vi "Menu.Sequeunce.Execute.vi"(8 "error in (no error)":errorcluster, 9 "Coords":T1, 10 "ItemPath":string, 11 "State Variables":T2={"Aliases.All"=[], "Aliases.Outputs"=[], "UI.Sequence#ofColumns"=0, "SysDef.Path"=path "", "UI.SequenceRef"=refnum, "UI.StepInformationRef"=refnum, "UI.AbortRef"=refnum, "UI.GraphRef"=refnum, "UI.ViewRef"=refnum, "UI.IterationsRef"=refnum, "UI.IterationInformationRef"=refnum, "INI.Settings"={"Build Location"=path "C:/Simple Sequence Editor/SequenceRepo", "LoggingLocation"=path ""}, "NIVS.Workspace Event"=refnum, "UI.SkipChannel"=refnum}) -> (0 "error out":errorcluster, 3 "State Variables out":T2={"Aliases.All"=[], "Aliases.Outputs"=[], "UI.Sequence#ofColumns"=0, "SysDef.Path"=path "", "UI.SequenceRef"=refnum, "UI.StepInformationRef"=refnum, "UI.AbortRef"=refnum, "UI.GraphRef"=refnum, "UI.ViewRef"=refnum, "UI.IterationsRef"=refnum, "UI.IterationInformationRef"=refnum, "INI.Settings"={"Build Location"=path "C:/Simple Sequence Editor/SequenceRepo", "LoggingLocation"=path ""}, "NIVS.Workspace Event"=refnum, "UI.SkipChannel"=refnum})   [LabVIEW 2013, in "Simple Sequence Tools - Editor.lvlib"]
uses:
  Simple Sequence Tools - Editor.lvlib
  Types/Main.StateVariables.ctl
  Shared/Types/Channel.Properties.ctl
  Shared/Types/INI.Settings
  <vilib>/Utility/miscctls.llb/LVPoint32TypeDef.ctl
  <vilib>/Utility/miscctls.llb/LVBoundsTypeDef.ctl
  Shared/SubVIs/Main.Constants.vi
  Shared/Simple Sequence Tools - Shared.lvlib
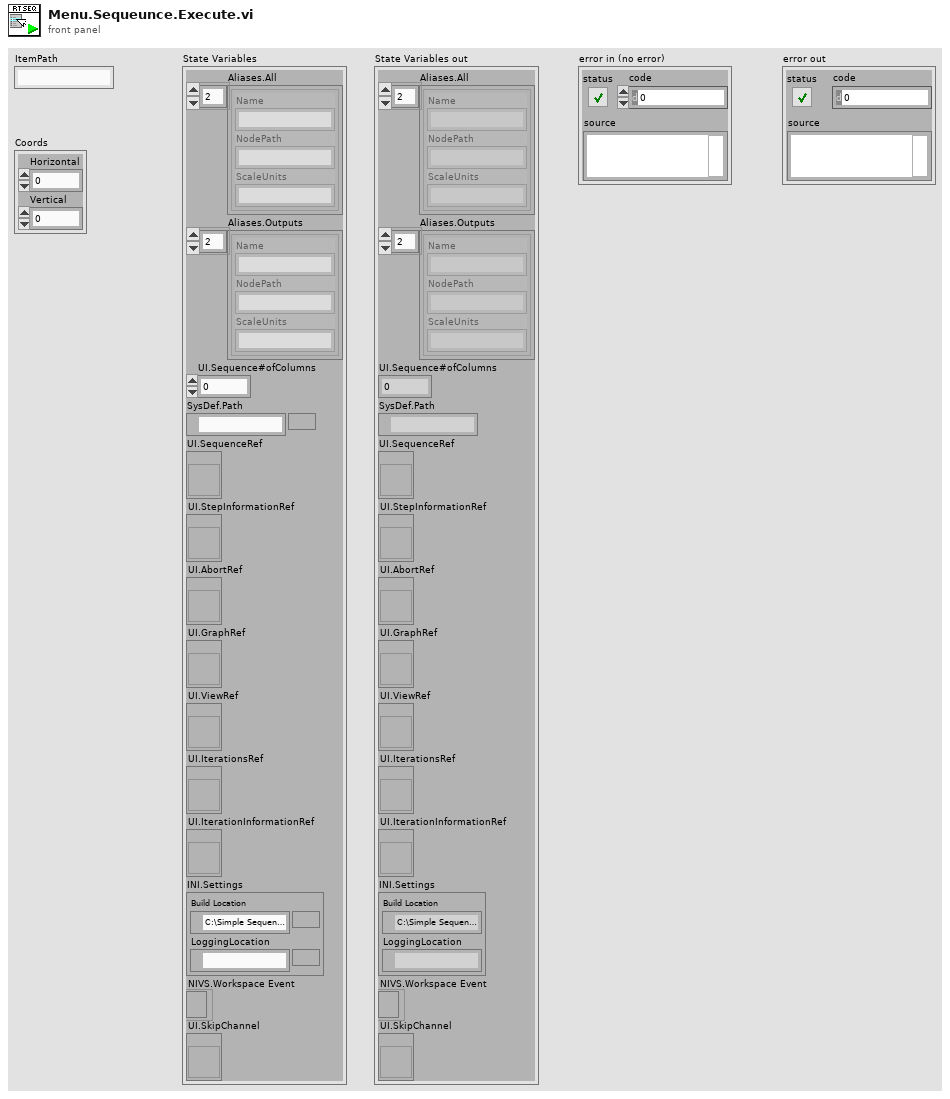
[diagram p1: front panel]
types:
  T1 = typedef "LVPoint32TypeDef.ctl" = cluster{"Horizontal":i32, "Vertical":i32}
  T2 = typedef "Simple Sequence Tools - Editor.lvlib/Main.StateVariables.ctl" = cluster{"Aliases.All":T3[], "Aliases.Outputs":T3[], "UI.Sequence#ofColumns":i32, "SysDef.Path":path, "UI.SequenceRef":refnum<vi>, "UI.StepInformationRef":refnum<vi>, "UI.AbortRef":refnum<vi>, "UI.GraphRef":refnum<vi>, "UI.ViewRef":refnum<vi>, "UI.IterationsRef":refnum<vi>, "UI.IterationInformationRef":refnum<vi>, "INI.Settings":T4, "NIVS.Workspace Event":refnum<event-registration>, "UI.SkipChannel":refnum<vi>}
  T3 = typedef "Simple Sequence Tools - Shared.lvlib/Channel.Properties.ctl" = cluster{"Name":string, "NodePath":string, "ScaleUnits":string}
  T4 = typedef "Simple Sequence Tools - Shared.lvlib/INI.Settings" = cluster{"Build Location":path, "LoggingLocation":path}
  T5 = typedef "LVRowAndColumnTypeDef.ctl" = cluster{"Row":i32, "Column":i32}
  T6 = typedef "LVBoundsTypeDef.ctl" = cluster{"Width":u32, "Height":u32}
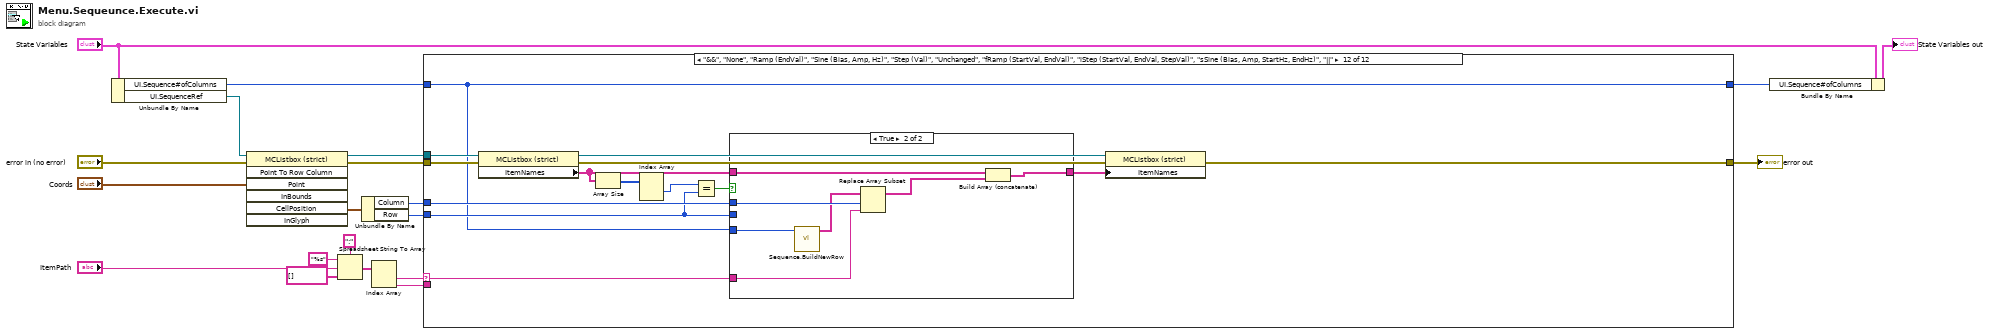
[diagram p0: block diagram]
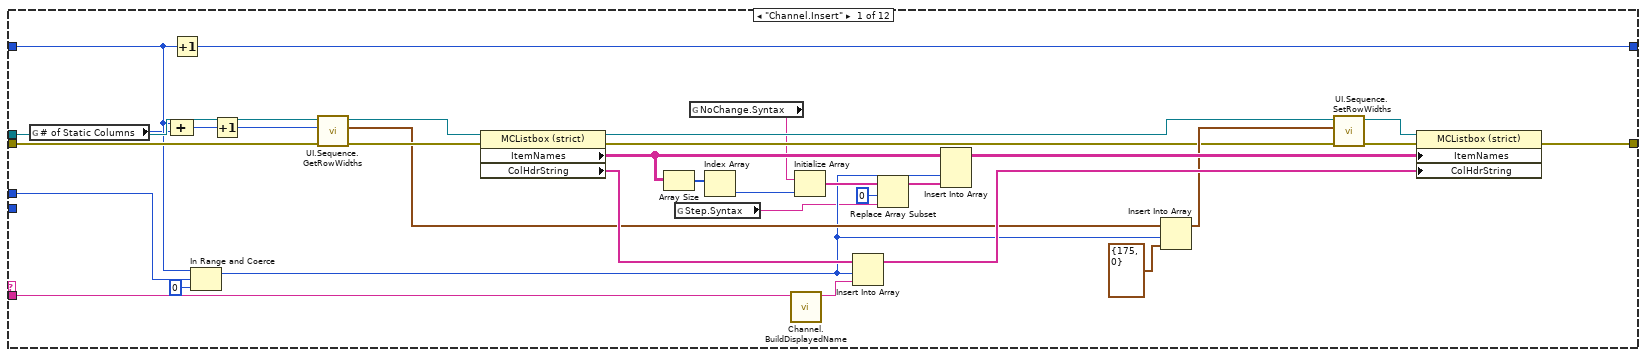
[diagram p2: hidden frame]
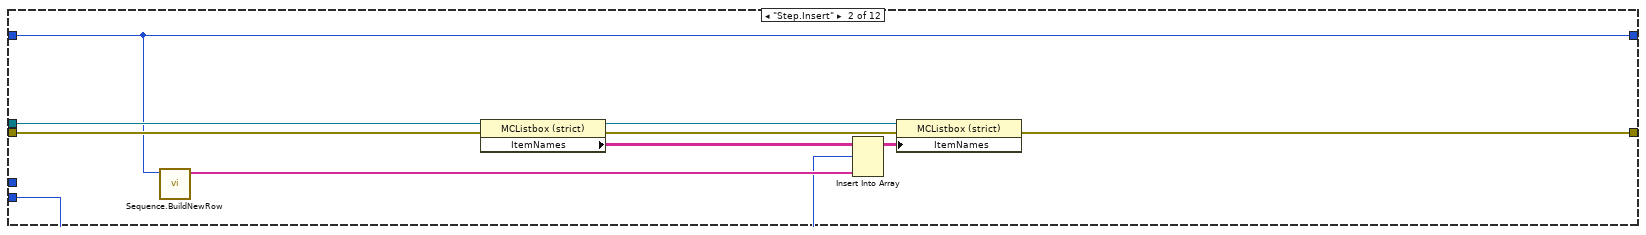
[diagram p3: hidden frame]
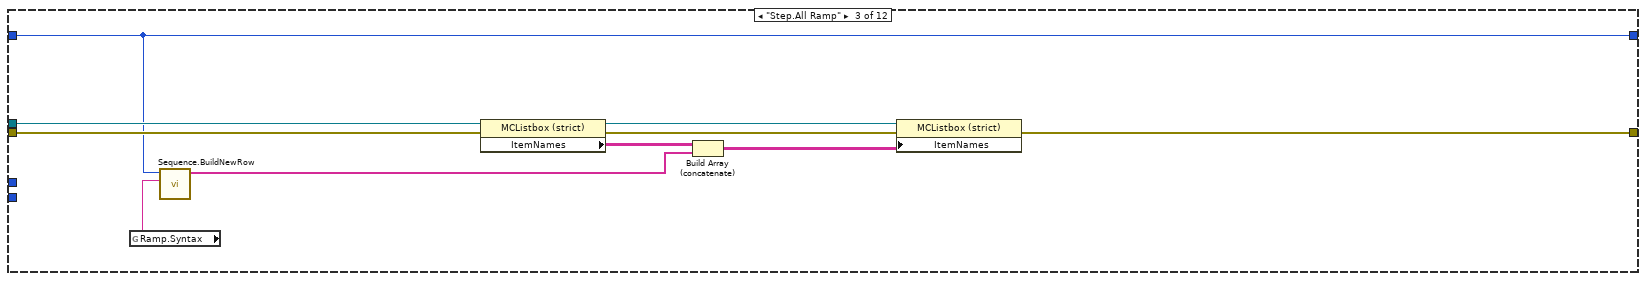
[diagram p4: hidden frame]
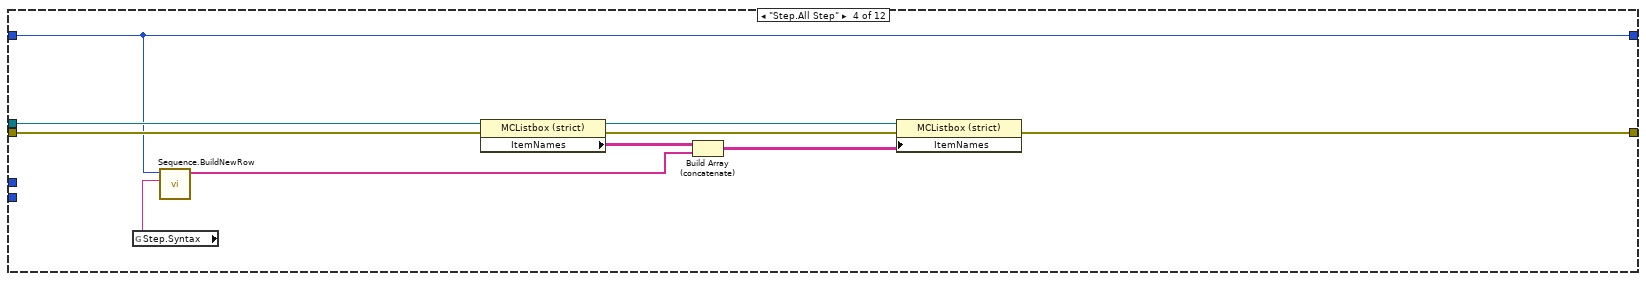
[diagram p5: hidden frame]
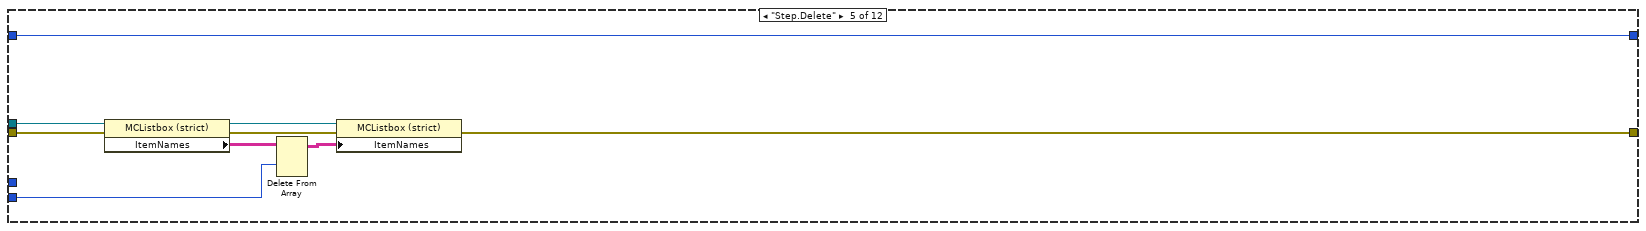
[diagram p6: hidden frame]
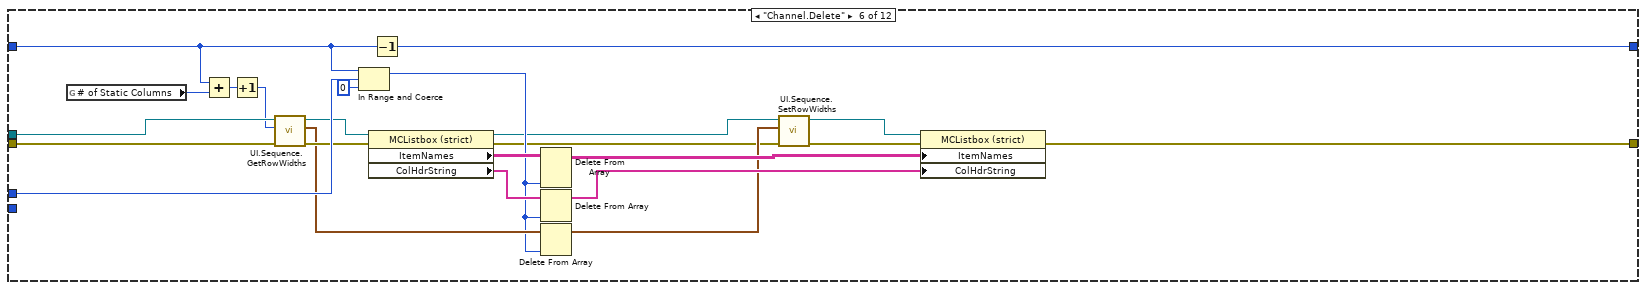
[diagram p7: hidden frame]
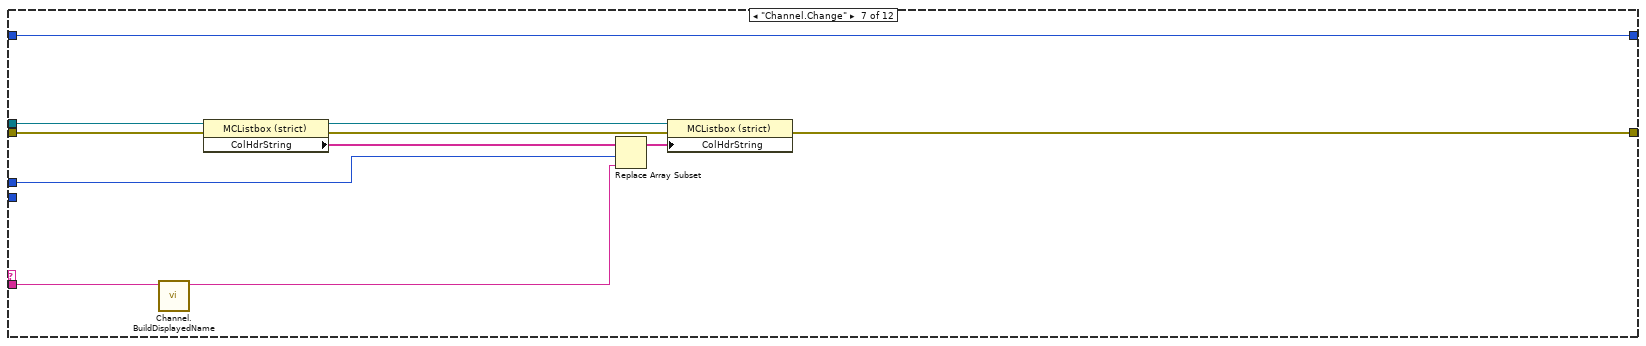
[diagram p8: hidden frame]
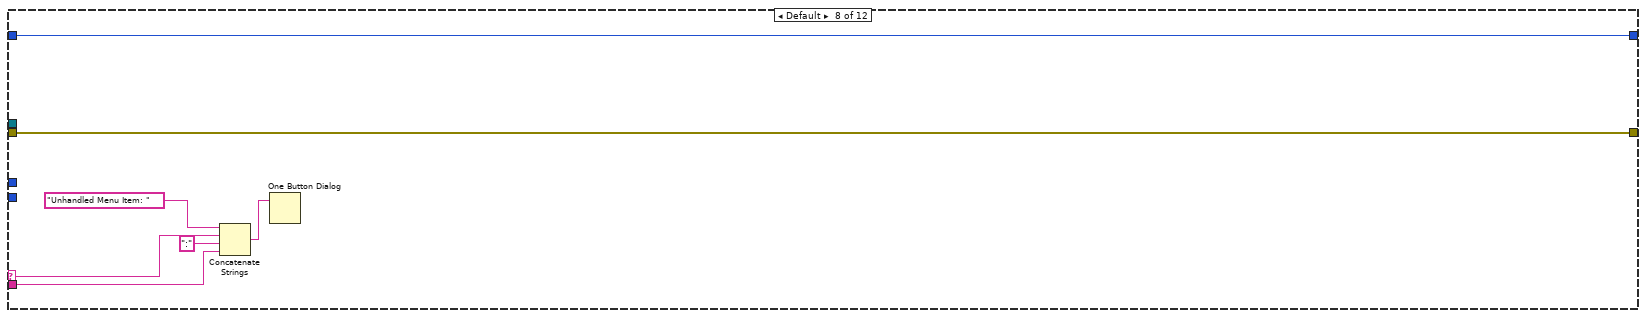
[diagram p9: hidden frame]
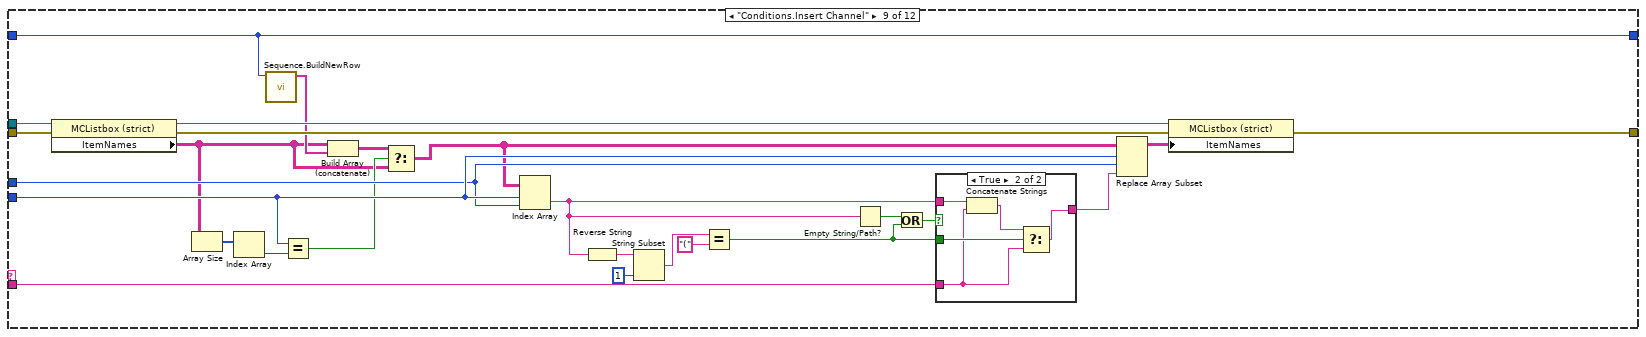
[diagram p10: hidden frame]
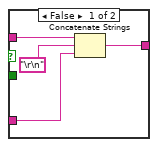
[diagram p11: hidden frame]
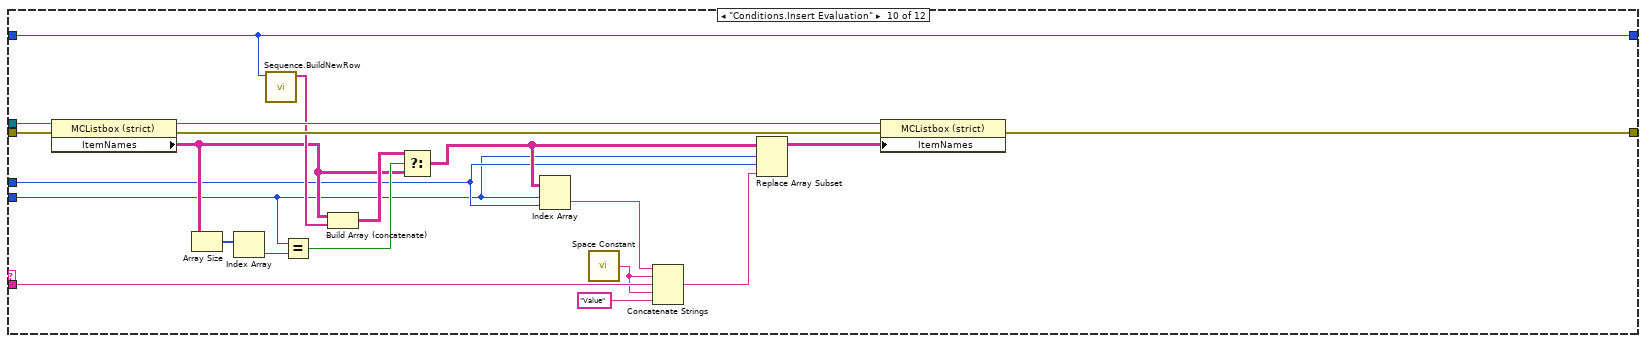
[diagram p12: hidden frame]
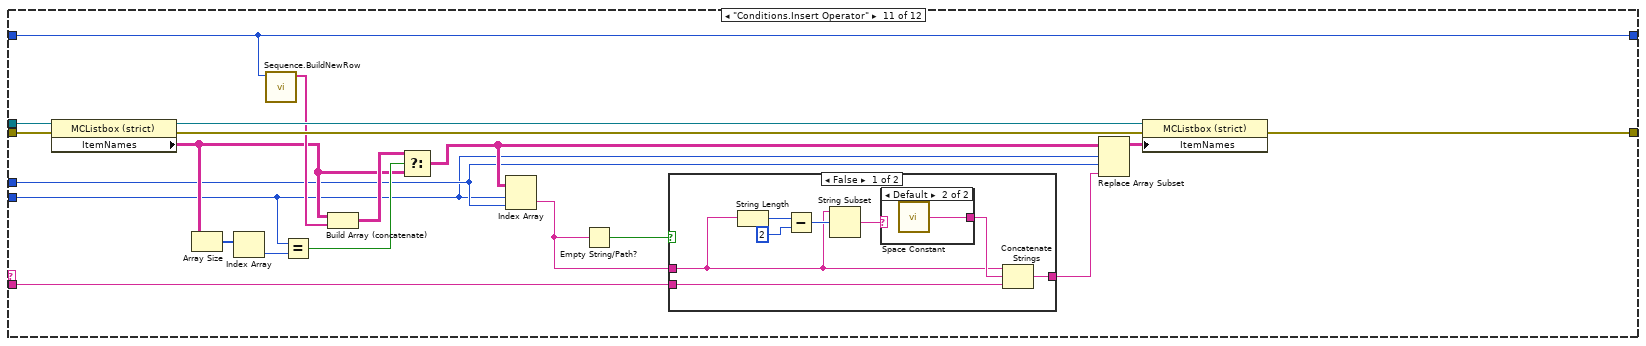
[diagram p13: hidden frame]
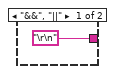
[diagram p14: hidden frame]
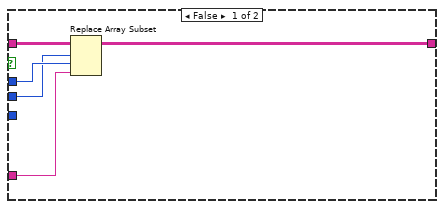
[diagram p16: hidden frame]
diagram:
  n1 = Unbundle By Name("State Variables") -> ("UI.Sequence#ofColumns"=w11:i32, "UI.SequenceRef"=w8:refnum<vi>)
  n2 = invoke class="MCListbox (strict)" method="Point To Row Column"(reference=w8, error in="error in (no error)", "Point"="Coords") -> (reference out=w13:refnum<vi>, error out=w14:errorcluster, "CellPosition"=w10:T5)  [unwired: 4 in, 4 out]
  n3 = Spreadsheet String To Array(delimiter (Tab)=":", format string="%s", spreadsheet string="ItemPath", array type (2D Dbl)=string[] []) -> (array=w6:string[])
  n4 = Unbundle By Name(w10) -> ("Column"=w12:i32, "Row"=w1:i32)
  n5 = Index Array(array=w6) -> (element #1=w7:string, element #2=w15:string)  [unwired: 2 in]
  n6 = case shown="\"&&\", \"None\", \"Ramp (EndVal)\", \"Sine (Bias, Amp, Hz)\", \"Step (Val)\", \"Unchanged\", \"fRamp (StartVal, EndVal)\", \"iStep (StartVal, EndVal, StepVal)\", \"sSine (Bias, Amp, StartHz, EndHz)\", \"||\"" w7 {
    selector: w7 -> [_ _ _ _ _ _ _ w131 _ _ _ w223]
    tunnel: w11 -> [w35 w54 w66 w76 w84 w99 w126 w133 w150 w182 w202 w221]
    tunnel: w12 -> [w53 _ _ _ _ w115 w119 _ w144 w172 w193 w229]
    tunnel: w13 -> [w38 w59 w69 w79 w88 w106 w120 _ w159 w189 w209 w233]
    tunnel: w14 -> [w40 w60 w70 w80 w89 w108 w121 w132 w158 w188 w208 w234]
    tunnel: w15 -> [w42 _ _ _ _ _ w117 w129 w154 w184 w204 _]
    tunnel: [w22 w61 w71 w81 w90 w93 w118 w132 w156 w186 w206 w222] -> w17
    tunnel: [w33 w54 w66 w76 w84 w113 w126 w133 w150 w182 w202 w221] -> w20
    tunnel: w1 -> [_ w55 _ _ w85 _ _ _ w147 w171 w192 w225]
    frame "Channel.Insert" {
      n7 = global read "Main.Constants.vi" "# of Static Columns"() -> (w34:u32)
      n8 = Compound Arithmetic op=ADD(w35, w34) -> (w36:u32)
      n9 = Increment(x=w35) -> (x+1=w33:i32)
      n10 = In Range and Coerce(upper limit=w35, x=w53, lower limit=0) -> (coerced(x)=w30:i32)  [unwired: 1 out]
      n11 = Increment(x=w36) -> (x+1=w28:u32)
      n12 = call "UI.Sequence.GetRowWidths.vi"("error in (no error)"=w40, "Numeric"=w28, "UI.SequenceRef"=w38) -> ("error out"=w39:errorcluster, "Array"=w31:T6[], "UI.SequenceRef"=w37:refnum<vi>)  [unwired: 6 in]
      n13 = property class="MCListbox (strict)"(reference=w37, error in=w39) -> (reference out=w23:refnum<vi>, error out=w26:errorcluster, "ItemNames"=w50:string[][], "ColHdrString"=w45:string[])
      n14 = Array Size(array=w50) -> (size(s)=w51:i32[])
      n15 = global read "Main.Constants.vi" "Step.Syntax"() -> (w27:string)
      n16 = global read "Main.Constants.vi" "NoChange.Syntax"() -> (w21:string)
      n17 = Index Array(array=w51) -> (element=w49:i32)  [unwired: 1 in]
      n18 = call "Channel.BuildDisplayedName.vi"("Path"=w42) -> ("Formated Path"=w41:string)  [unwired: 10 in]
      n19 = Initialize Array(w21, w49) -> (w48:string[])
      n20 = Insert Into Array(array=w45, index=w30, new element=w41) -> (w46:string[])
      n21 = Replace Array Subset(array=w48, new element=w27, index=0) -> (w44:string[])
      n22 = Insert Into Array(array=w50, index (col)=w30, new element=w44) -> (w47:string[][])  [unwired: 1 in]
      n23 = Insert Into Array(array=w31, index=w30, new element=T6 {"Width"=175, "Height"=0} ("new element/subarray")) -> (w32:T6[])
      n24 = call "UI.Sequence.SetRowWidths.vi"("error in (no error)"=w26, "CellSize"=w32, "UI.SequenceRef"=w23) -> ("error out"=w25:errorcluster, "UI.SequenceRef"=w24:refnum<vi>)  [unwired: 7 in]
      n25 = property class="MCListbox (strict)"(reference=w24, error in=w25, "ItemNames"=w47, "ColHdrString"=w46) -> (error out=w22:errorcluster)  [unwired: 1 out]
    }
    frame "Step.Insert" {
      n26 = call "Sequence.BuildNewRow.vi"("UI.Sequence#ofColumns"=w54) -> ("New Array"=w58:string[])  [unwired: 10 in]
      n27 = property class="MCListbox (strict)"(reference=w59, error in=w60) -> (reference out=w56:refnum<vi>, error out=w57:errorcluster, "ItemNames"=w63:string[][])
      n28 = Insert Into Array(array=w63, index (row)=w55, new element=w58) -> (w62:string[][])  [unwired: 1 in]
      n29 = property class="MCListbox (strict)"(reference=w56, error in=w57, "ItemNames"=w62) -> (error out=w61:errorcluster)  [unwired: 1 out]
    }
    frame "Step.All Ramp" {
      n30 = global read "Main.Constants.vi" "Ramp.Syntax"() -> (w65:string)
      n31 = call "Sequence.BuildNewRow.vi"("Syntax"=w65, "UI.Sequence#ofColumns"=w66) -> ("New Array"=w64:string[])  [unwired: 9 in]
      n32 = property class="MCListbox (strict)"(reference=w69, error in=w70) -> (reference out=w67:refnum<vi>, error out=w68:errorcluster, "ItemNames"=w73:string[][])
      n33 = Build Array (concatenate)(w73, w64) -> (w72:string[][])
      n34 = property class="MCListbox (strict)"(reference=w67, error in=w68, "ItemNames"=w72) -> (error out=w71:errorcluster)  [unwired: 1 out]
    }
    frame "Step.All Step" {
      n35 = global read "Main.Constants.vi" "Step.Syntax"() -> (w75:string)
      n36 = call "Sequence.BuildNewRow.vi"("Syntax"=w75, "UI.Sequence#ofColumns"=w76) -> ("New Array"=w74:string[])  [unwired: 9 in]
      n37 = property class="MCListbox (strict)"(reference=w79, error in=w80) -> (reference out=w77:refnum<vi>, error out=w78:errorcluster, "ItemNames"=w83:string[][])
      n38 = Build Array (concatenate)(w83, w74) -> (w82:string[][])
      n39 = property class="MCListbox (strict)"(reference=w77, error in=w78, "ItemNames"=w82) -> (error out=w81:errorcluster)  [unwired: 1 out]
    }
    frame "Step.Delete" {
      n40 = property class="MCListbox (strict)"(reference=w88, error in=w89) -> (reference out=w86:refnum<vi>, error out=w87:errorcluster, "ItemNames"=w92:string[][])
      n41 = Delete From Array(array=w92, index (row)=w85) -> (array with subset deleted=w91:string[][])  [unwired: 2 in, 1 out]
      n42 = property class="MCListbox (strict)"(reference=w86, error in=w87, "ItemNames"=w91) -> (error out=w90:errorcluster)  [unwired: 1 out]
    }
    frame "Channel.Delete" {
      n43 = global read "Main.Constants.vi" "# of Static Columns"() -> (w101:u32)
      n44 = Add(x=w99, y=w101) -> (x+y=w100:u32)
      n45 = Increment(x=w100) -> (x+1=w98:u32)
      n46 = call "UI.Sequence.GetRowWidths.vi"("error in (no error)"=w108, "Numeric"=w98, "UI.SequenceRef"=w106) -> ("error out"=w107:errorcluster, "Array"=w104:T6[], "UI.SequenceRef"=w105:refnum<vi>)  [unwired: 6 in]
      n47 = In Range and Coerce(upper limit=w99, x=w115, lower limit=0) -> (coerced(x)=w103:i32)  [unwired: 1 out]
      n48 = property class="MCListbox (strict)"(reference=w105, error in=w107) -> (reference out=w94:refnum<vi>, error out=w97:errorcluster, "ItemNames"=w112:string[][], "ColHdrString"=w109:string[])
      n49 = Decrement(x=w99) -> (x-1=w113:i32)
      n50 = Delete From Array(array=w112, index (col)=w103) -> (array with subset deleted=w111:string[][])  [unwired: 2 in, 1 out]
      n51 = Delete From Array(array=w109, index=w103) -> (array with subset deleted=w110:string[])  [unwired: 1 in, 1 out]
      n52 = Delete From Array(array=w104, index=w103) -> (array with subset deleted=w102:T6[])  [unwired: 1 in, 1 out]
      n53 = call "UI.Sequence.SetRowWidths.vi"("error in (no error)"=w97, "CellSize"=w102, "UI.SequenceRef"=w94) -> ("error out"=w96:errorcluster, "UI.SequenceRef"=w95:refnum<vi>)  [unwired: 7 in]
      n54 = property class="MCListbox (strict)"(reference=w95, error in=w96, "ItemNames"=w111, "ColHdrString"=w110) -> (error out=w93:errorcluster)  [unwired: 1 out]
    }
    frame "Channel.Change" {
      n55 = call "Channel.BuildDisplayedName.vi"("Path"=w117) -> ("Formated Path"=w116:string)  [unwired: 10 in]
      n56 = property class="MCListbox (strict)"(reference=w120, error in=w121) -> (reference out=w125:refnum<vi>, error out=w124:errorcluster, "ColHdrString"=w122:string[])
      n57 = Replace Array Subset(array=w122, new element=w116, index=w119) -> (w123:string[])
      n58 = property class="MCListbox (strict)"(reference=w125, error in=w124, "ColHdrString"=w123) -> (error out=w118:errorcluster)  [unwired: 1 out]
    }
    frame Default {
      n59 = Concatenate Strings("Unhandled Menu Item: " ("message"), w131, ":" ("string"), w129) -> (w127:string)
      n60 = One Button Dialog(message=w127) -> ()  [unwired: 1 in, 1 out]
    }
    frame "Conditions.Insert Channel" {
      n61 = property class="MCListbox (strict)"(reference=w159, error in=w158) -> (reference out=w155:refnum<vi>, error out=w157:errorcluster, "ItemNames"=w142:string[][])
      n62 = Array Size(array=w142) -> (size(s)=w149:i32[])
      n63 = Index Array(array=w149) -> (element=w148:i32)  [unwired: 1 in]
      n64 = call "Sequence.BuildNewRow.vi"("UI.Sequence#ofColumns"=w150) -> ("New Array"=w146:string[])  [unwired: 10 in]
      n65 = Equal?(x=w147, y=w148) -> (x = y?=w143:bool)
      n66 = Build Array (concatenate)(w142, w146) -> (w145:string[][])
      n67 = Select(t=w145, s=w143, f=w142) -> (s? t:f=w139:string[][])
      n68 = Index Array(array=w139, index (row)=w147, index (col)=w144) -> (element=w135:string)
      n69 = Reverse String(1:w135) -> (0:w137:string)
      n70 = String Subset(string=w137, length (rest)=1 ("length (rest)")) -> (substring=w134:string)  [unwired: 1 in]
      n71 = Equal?(x=w134, y="(") -> (x = y?=w138:bool)
      n72 = Empty String/Path?(string/path=w135) -> (empty?=w153:bool)
      n73 = Or(x=w153, y=w138) -> (x .or. y?=w140:bool)
      n74 = case shown="True" w140 {
        tunnel: w135 -> [w163 w167]
        tunnel: w154 -> [w162 w166]
        tunnel: [w160 w165] -> w152
        tunnel: w138 -> [_ w168]
        frame False {
          n75 = Concatenate Strings(w163, "\r\n", w162) -> (w160:string)
        }
        frame True {
          n76 = Concatenate Strings(w167, w166) -> (w164:string)
          n77 = Select(t=w164, s=w168, f=w166) -> (s? t:f=w165:string)
        }
      }
      n78 = Replace Array Subset(array=w139, new element=w152, index (row)=w147, index (col)=w144) -> (w151:string[][])
      n79 = property class="MCListbox (strict)"(reference=w155, error in=w157, "ItemNames"=w151) -> (error out=w156:errorcluster)  [unwired: 1 out]
    }
    frame "Conditions.Insert Evaluation" {
      n80 = property class="MCListbox (strict)"(reference=w189, error in=w188) -> (reference out=w185:refnum<vi>, error out=w187:errorcluster, "ItemNames"=w176:string[][])
      n81 = Array Size(array=w176) -> (size(s)=w181:i32[])
      n82 = Index Array(array=w181) -> (element=w180:i32)  [unwired: 1 in]
      n83 = call "Sequence.BuildNewRow.vi"("UI.Sequence#ofColumns"=w182) -> ("New Array"=w179:string[])  [unwired: 10 in]
      n84 = Equal?(x=w171, y=w180) -> (x = y?=w177:bool)
      n85 = Build Array (concatenate)(w176, w179) -> (w178:string[][])
      n86 = Select(t=w178, s=w177, f=w176) -> (s? t:f=w173:string[][])
      n87 = Index Array(array=w173, index (row)=w171, index (col)=w172) -> (element=w169:string)
      n88 = call <vilib>:"Space Constant.vi"() -> ("String"=w170:string)
      n89 = Concatenate Strings(w169, w170, w184, w170, "Value" ("string")) -> (w175:string)
      n90 = Replace Array Subset(array=w173, new element=w175, index (row)=w171, index (col)=w172) -> (w183:string[][])
      n91 = property class="MCListbox (strict)"(reference=w185, error in=w187, "ItemNames"=w183) -> (error out=w186:errorcluster)  [unwired: 1 out]
    }
    frame "Conditions.Insert Operator" {
      n92 = property class="MCListbox (strict)"(reference=w209, error in=w208) -> (reference out=w205:refnum<vi>, error out=w207:errorcluster, "ItemNames"=w196:string[][])
      n93 = Array Size(array=w196) -> (size(s)=w201:i32[])
      n94 = Index Array(array=w201) -> (element=w200:i32)  [unwired: 1 in]
      n95 = call "Sequence.BuildNewRow.vi"("UI.Sequence#ofColumns"=w202) -> ("New Array"=w199:string[])  [unwired: 10 in]
      n96 = Equal?(x=w192, y=w200) -> (x = y?=w197:bool)
      n97 = Build Array (concatenate)(w196, w199) -> (w198:string[][])
      n98 = Select(t=w198, s=w197, f=w196) -> (s? t:f=w194:string[][])
      n99 = Index Array(array=w194, index (row)=w192, index (col)=w193) -> (element=w191:string)
      n100 = Empty String/Path?(string/path=w191) -> (empty?=w190:bool)
      n101 = case shown="False" w190 {
        tunnel: w204 -> [w217 w220]
        tunnel: [w216 w220] -> w195
        tunnel: w191 -> [w210 _]
        frame False {
          n102 = String Length(string=w210) -> (length=w215:i32)
          n103 = Subtract(x=w215, y=2) -> (x-y=w214:i32)
          n104 = String Subset(string=w210, offset (0)=w214) -> (substring=w212:string)  [unwired: 1 in]
          n105 = case shown="Default" w212 {
            tunnel: ["\r\n" w219] -> w211
            frame "&&", "||" {
            }
            frame Default {
              n106 = call <vilib>:"Space Constant.vi"() -> ("String"=w219:string)
            }
          }
          n107 = Concatenate Strings(w210, w211, w217) -> (w216:string)
        }
        frame True {
        }
      }
      n108 = Replace Array Subset(array=w194, new element=w195, index (row)=w192, index (col)=w193) -> (w203:string[][])
      n109 = property class="MCListbox (strict)"(reference=w205, error in=w207, "ItemNames"=w203) -> (error out=w206:errorcluster)  [unwired: 1 out]
    }
    frame "&&", "None", "Ramp (EndVal)", "Sine (Bias, Amp, Hz)", "Step (Val)", "Unchanged", "fRamp (StartVal, EndVal)", "iStep (StartVal, EndVal, StepVal)", "sSine (Bias, Amp, StartHz, EndHz)", "||" {
      n110 = property class="MCListbox (strict)"(reference=w233, error in=w234) -> (reference out=w231:refnum<vi>, error out=w232:errorcluster, "ItemNames"=w228:string[][])
      n111 = Array Size(array=w228) -> (size(s)=w227:i32[])
      n112 = Index Array(array=w227) -> (element #1=w226:i32)  [unwired: 2 in, 1 out]
      n113 = Equal?(x=w226, y=w225) -> (x = y?=w224:bool)
      n114 = case shown="True" w224 {
        tunnel: [w239 w245] -> w230
        tunnel: w229 -> [w238 w244]
        tunnel: w228 -> [w237 w246]
        tunnel: w225 -> [w236 _]
        tunnel: w221 -> [_ w241]
        tunnel: w223 -> [w235 w243]
        frame False {
          n115 = Replace Array Subset(array=w237, new element=w235, index (row)=w236, index (col)=w238) -> (w239:string[][])
        }
        frame True {
          n116 = call "Sequence.BuildNewRow.vi"("UI.Sequence#ofColumns"=w241) -> ("New Array"=w240:string[])  [unwired: 10 in]
          n117 = Replace Array Subset(array=w240, new element=w243, index=w244) -> (w242:string[])
          n118 = Build Array (concatenate)(w246, w242) -> (w245:string[][])
        }
      }
      n119 = property class="MCListbox (strict)"(reference=w231, error in=w232, "ItemNames"=w230) -> (error out=w222:errorcluster)  [unwired: 1 out]
    }
  }
  "error out" <- w17
  n120 = Bundle By Name(cluster="State Variables", "UI.Sequence#ofColumns"=w20) -> (→"State Variables out":T2)
